vi "DIAGNOSTICO.vi"() -> ()   [LabVIEW 2024]
uses:
  <vilib>/numeric/Random Number (Range) DBL.vi
panel:
  out "concatenated string":string
  out "Dentro":bool
  in  "stop":bool
  out "histeresis":bool
  out "Waveform Chart":dynamicdata(graph)
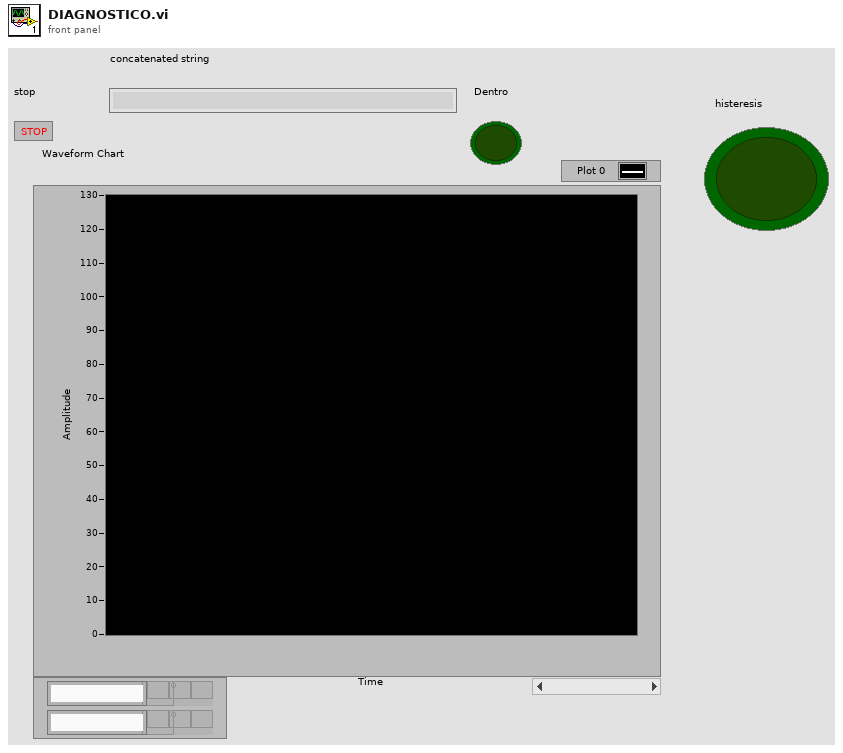
[diagram p1: front panel]
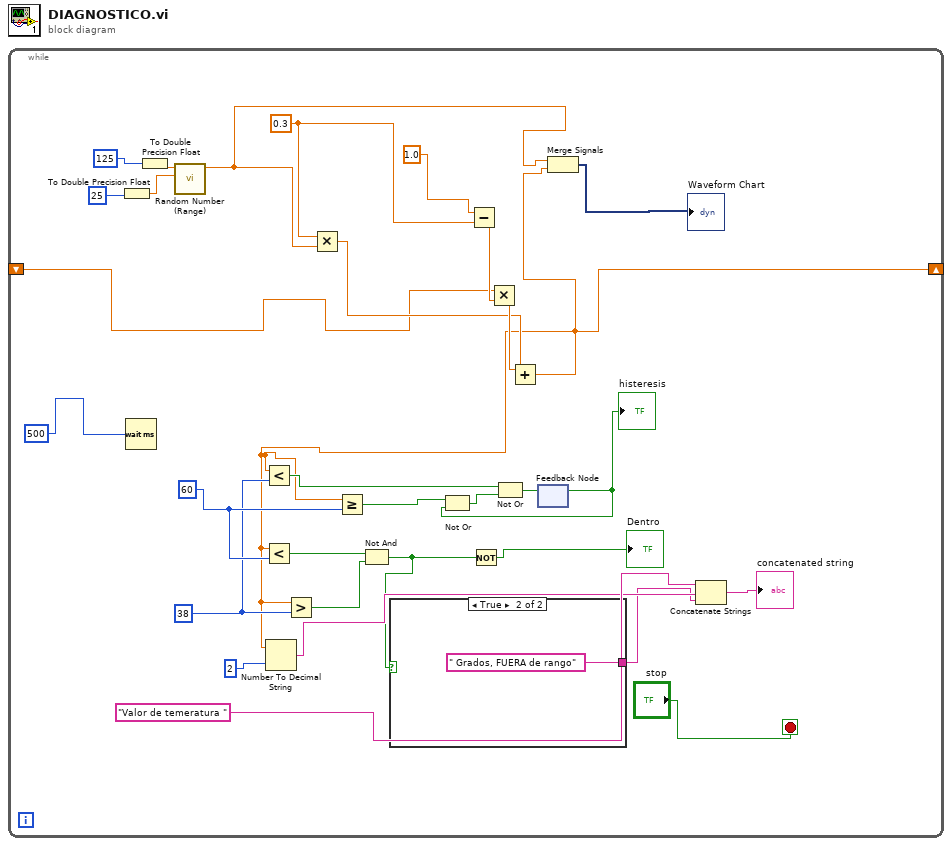
[diagram p0: block diagram]
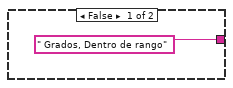
[diagram p2: hidden frame]
diagram:
  n1 = while {
    shift-right: [w8] -> _
    shift-left: _ -> [w26]
    stop <- "stop" stop-if-true
    w13 = 38
    w17 = 60
    w30 = 0.3
    n2 = To Double Precision Float(number=25) -> (double precision float=w20:dbl)
    n3 = Wait (ms)(milliseconds to wait=500) -> ()  [unwired: 1 out]
    n4 = To Double Precision Float(number=125) -> (double precision float=w22:dbl)
    n5 = call-poly <vilib>:"Random Number (Range).vi"("lower bound (0)"=w20, "upper bound (100)"=w22) -> ("number"=w24:dbl)  [unwired: 9 in]
    n6 = Multiply(x=w30, y=w24) -> (x*y=w27:dbl)
    n7 = Subtract(x=1.0, y=w30) -> (x-y=w29:dbl)
    n8 = Multiply(x=w26, y=w29) -> (x*y=w28:dbl)
    n9 = Add(x=w28, y=w27) -> (x+y=w8:dbl)
    n10 = Less?(x=w8, y=w13) -> (x < y?=w11:bool)
    n11 = Less?(x=w8, y=w17) -> (x < y?=w15:bool)
    n12 = Number To Decimal String(number=w8, width (-)=2) -> (decimal integer string=w5:string)
    n13 = Greater?(x=w8, y=w13) -> (0:w14:bool)
    n14 = Greater Or Equal?(x=w8, y=w17) -> (x >= y?=w16:bool)
    n15 = Not And(1:w14, 2:w15) -> (0:w2:bool)
    n16 = case shown="True" w2 {
      tunnel: [" Grados, Dentro de rango" " Grados, FUERA de rango"] -> w4
      frame False {
      }
      frame True {
      }
    }
    n17 = Not(x=w2) -> (.not. x?=→"Dentro":bool)
    n18 = feedback #1() -> (w9:bool)  [unwired: 1 in]
    "histeresis" <- w9
    n19 = Not Or(1:w9, 2:w16) -> (0:w12:bool)
    n20 = Not Or(1:w12, 2:w11) -> (0:w10:bool)
    n21 = feedback-in #1(w10) -> ()
    n22 = Merge Signals(w24, w8) -> (→"Waveform Chart":dynamicdata)
    n23 = Concatenate Strings("Valor de temeratura ", w5, w4) -> (→"concatenated string":string)
  }
